vi "Get Power as Percentage.vi"(0 "COM Port in":refnum<visa-resource-name>, 1 "error in":errorcluster) -> (2 "COM Port out":refnum<visa-resource-name>, 3 "power value":dbl, 4 "OK":bool, 5 "error out":errorcluster)   [LabVIEW 2015]
doc: "This command determines the actual stored set point value for the optical laser/led power."
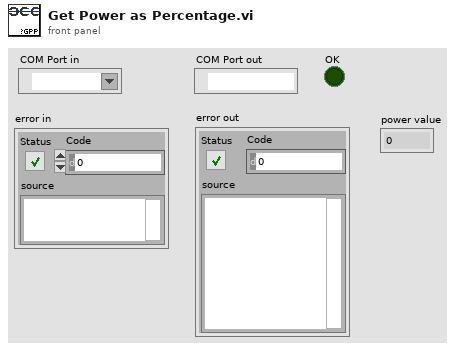
[diagram p1: front panel]
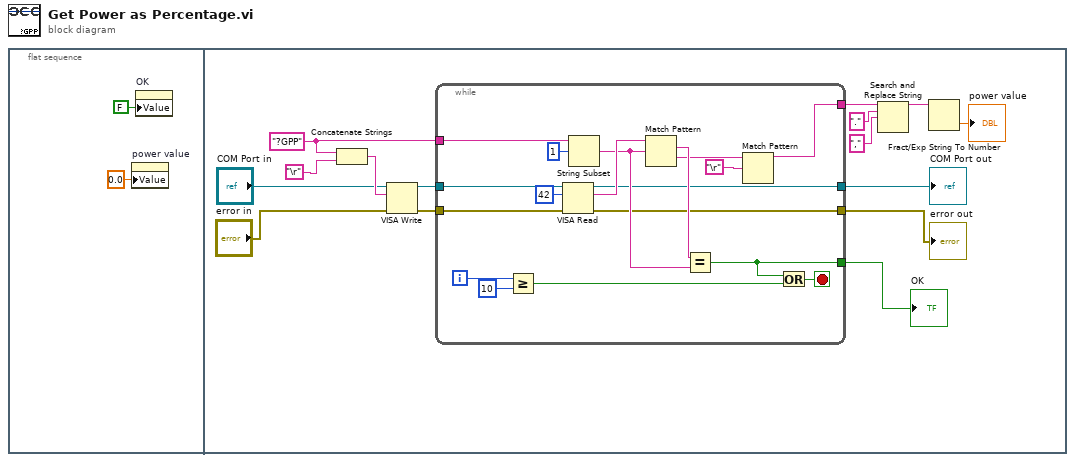
[diagram p0: block diagram]
diagram:
  n1 = flat-sequence {
    frame #0 {
      n2 = property on="power value" class="DigNum (strict)"("Value"=0.0 ("power value")) -> ()  [unwired: 2 in, 2 out]
      n3 = property on="OK" class="Bool (strict)"("Value"=FALSE ("OK")) -> ()  [unwired: 2 in, 2 out]
    }
    frame #1 {
      w11 = "?GPP" ("Schreibpuffer")
      n4 = Concatenate Strings(w11, "\r") -> (w15:string)
      n5 = VISA Write(VISA resource name="COM Port in", write buffer=w15, error in (no error)="error in") -> (VISA resource name out=w13:refnum<visa-resource-name>, error out=w12:errorcluster)  [unwired: 1 out]
      n6 = while {
        tunnel: [w30] -> w17
        tunnel: [w29] -> w16
        tunnel: [w25] -> w6
        tunnel: w13 -> [w19]
        tunnel: w12 -> [w22]
        tunnel: w11 -> [w21]
        tunnel: [w20] -> w8
        i -> [w28]
        stop <- w23 stop-if-true
        n7 = Greater Or Equal?(x=w28, y=10) -> (x >= y?=w26:bool)
        n8 = VISA Read(VISA resource name=w19, byte count=u32 42 ("Byte-Anzahl"), error in (no error)=w22) -> (VISA resource name out=w30:refnum<visa-resource-name>, read buffer=w34:string, error out=w29:errorcluster)  [unwired: 1 out]
        n9 = String Subset(string=w21, offset (0)=1 ("Offset (0)")) -> (substring=w31:string)  [unwired: 1 in]
        n10 = Match Pattern(string=w34, regular expression=w31) -> (match substring=w33:string, after substring=w24:string)  [unwired: 1 in, 2 out]
        n11 = Equal?(x=w33, y=w31) -> (x = y?=w20:bool)
        n12 = Match Pattern(string=w24, regular expression="\r") -> (before substring=w25:string)  [unwired: 1 in, 3 out]
        n13 = Or(x=w20, y=w26) -> (x .or. y?=w23:bool)
      }
      "COM Port out" <- w17
      "error out" <- w16
      "OK" <- w8
      n14 = Search and Replace String(input string=w6, search string="." ("Such-String"), replace string="," ("String ersetzen(\"\")")) -> (result string=w5:string)  [unwired: 5 in, 3 out]
      n15 = Fract/Exp String To Number(string=w5) -> (number=→"power value":dbl)  [unwired: 3 in, 1 out]
    }
  }
